vi "SectionA04_Week5_Stus.vi"() -> ()   [LabVIEW 2013]
uses:
  <vilib>/measure/mascope.llb/Amplitude and Levels 1 chan.vi
  <vilib>/measure/NI_MAPro.lvlib
panel:
  out "Peak-to-Peak Voltage Inverting Opamp":dbl
  out "Peak-to-Peak Voltage Non-Inverting Opamp":dbl
  out "Peak-to-Peak Voltage of Input":dbl
  out "Waveform Graph":dbl[][](graph)
  in  "Gain":dbl
  in  "Frequency of Input (mHz)":dbl
  in  "Peak Voltage of Input":dbl
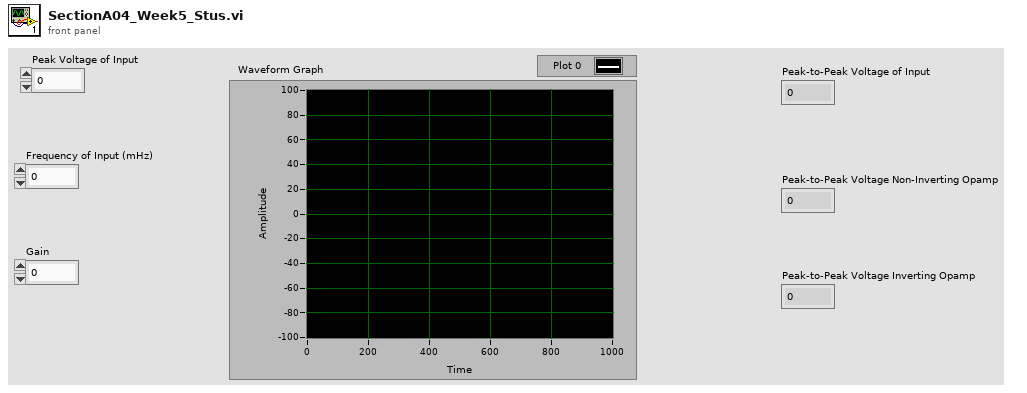
[diagram p1: front panel]
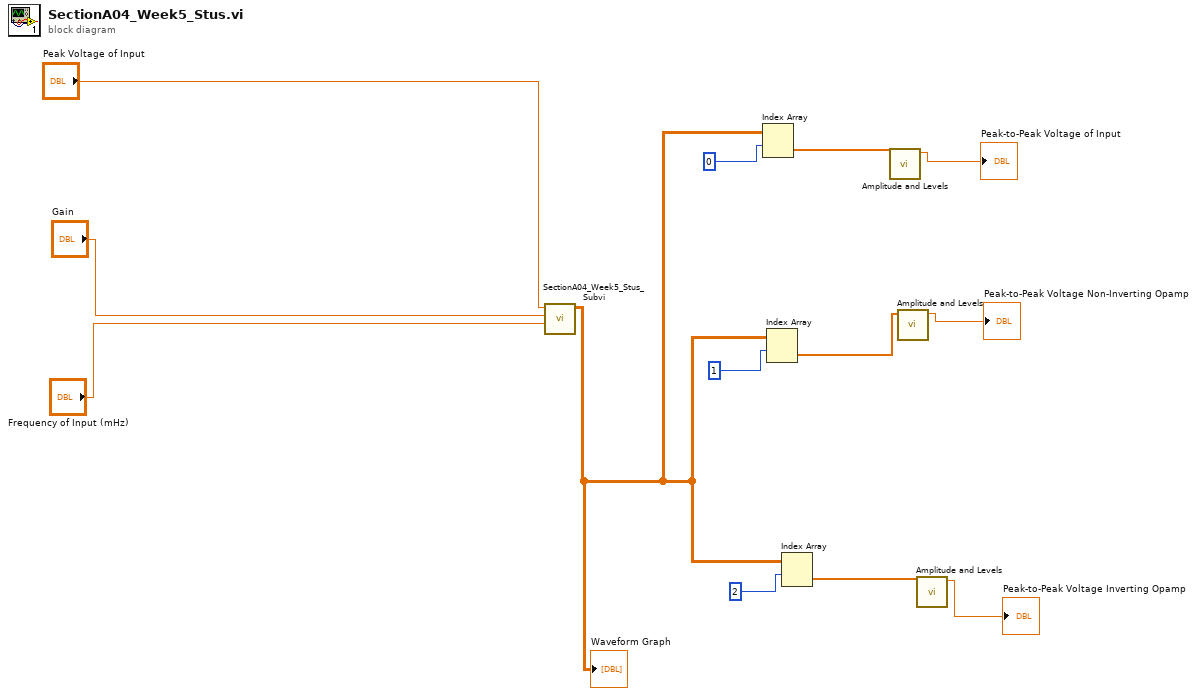
[diagram p0: block diagram]
diagram:
  n1 = call "SectionA04_Week5_Stus_Subvi.vi"("Frequency of Input (mHz)"="Frequency of Input (mHz)", "Gain"="Gain", "Peak Voltage of Input"="Peak Voltage of Input") -> ("Array"=w2:dbl[][])  [unwired: 8 in]
  "Waveform Graph" <- w2
  n2 = Index Array(array=w2, index (row)=0) -> (element=w5:dbl[])  [unwired: 1 in]
  n3 = Index Array(array=w2, index (row)=1) -> (element=w4:dbl[])  [unwired: 1 in]
  n4 = Index Array(array=w2, index (row)=2) -> (element=w3:dbl[])  [unwired: 1 in]
  n5 = call-poly <vilib>:"Amplitude and Levels.vi"("signal in"=w5) -> ("amplitude"=→"Peak-to-Peak Voltage of Input":dbl)  [unwired: 7 in, 3 out]
  n6 = call-poly <vilib>:"Amplitude and Levels.vi"("signal in"=w4) -> ("amplitude"=→"Peak-to-Peak Voltage Non-Inverting Opamp":dbl)  [unwired: 7 in, 3 out]
  n7 = call-poly <vilib>:"Amplitude and Levels.vi"("signal in"=w3) -> ("amplitude"=→"Peak-to-Peak Voltage Inverting Opamp":dbl)  [unwired: 7 in, 3 out]
